vi "GetSetMatchInterval.vi"(8 "error in":errorcluster, 9 "Match interval":u16 max=300 step=1, 10 "get/set":T1, 11 "VISA resource name":refnum<visa-resource-name>) -> (0 "error out":errorcluster, 2 "Service request interval":string, 3 "VISA resource name out":refnum<visa-resource-name>)   [LabVIEW 2023, in "Thermotron 8800.lvlib"]
doc: "MINT\nCommand name: Send or load match interval\nCommand type: System status\nDescription: The match interval is used to trigger the interval match interrupt event for a service request. The interval match interrupt event occurs at the beginning of the previously loaded match interval. If the value loaded for the match interval is 0, the match interval event will occur at the beginning of every interval.\nSyntax: MINT? or MINTdata\nData type: Integer (range 0 to 300)\nQuery example: MINT?\n8800 response: 14 (A service request interrupt will occur at the start of interval 14 when running a program.)\nOperation example: MINT3\n8800 response: The 8800 loads the match interval parameter with a value of 3."
uses:
  Thermotron 8800.lvlib
  Private/get set.ctl
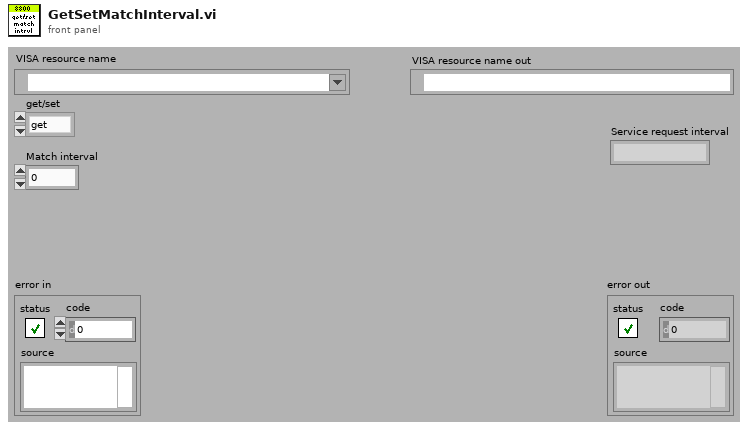
[diagram p1: front panel]
types:
  T1 = typedef "Thermotron 8800.lvlib/get set.ctl" = enum16{"get", "set"}
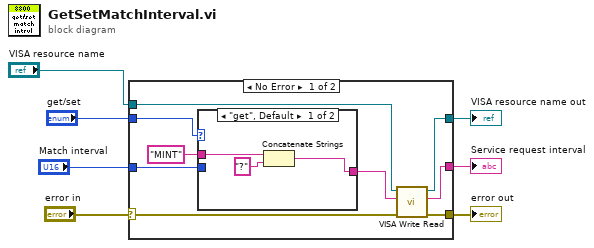
[diagram p0: block diagram]
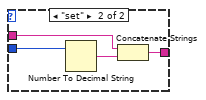
[diagram p2: hidden frame]
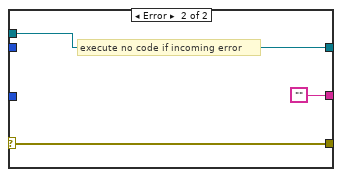
[diagram p3: hidden frame]
diagram:
  n1 = case shown="No Error" "error in" {
    selector: "error in" -> [w8 w25]
    tunnel: "get/set" -> [w16 _]
    tunnel: [w13 ""] -> w1
    tunnel: [w12 w25] -> w4
    tunnel: [w11 w26] -> w6
    tunnel: "VISA resource name" -> [w10 w26]
    tunnel: "Match interval" -> [w9 _]
    frame No Error {
      n2 = case shown="\"get\", Default" w16 {
        tunnel: "MINT" ("8800 Command") -> [w18 w23]
        tunnel: [w19 w22] -> w14
        tunnel: w9 -> [_ w20]
        frame "get", Default {
          n3 = Concatenate Strings(w18, "?" ("8800 Command")) -> (w19:string)
        }
        frame "set" {
          n4 = Number To Decimal String(number=w20) -> (decimal integer string=w21:string)  [unwired: 1 in]
          n5 = Concatenate Strings(w23, w21) -> (w22:string)
        }
      }
      n6 = call "VISA Write Read.vi"("error in (no error)"=w8, "8800 Command"=w14, "VISA Refnum in"=w10) -> ("error out"=w12:errorcluster, "read buffer"=w13:string, "VISA Refnum out"=w11:refnum<visa-resource-name>)  [unwired: 6 in]
    }
    frame Error {
      # "execute no code if incoming error"
    }
  }
  "VISA resource name out" <- w6
  "error out" <- w4
  "Service request interval" <- w1
